vi "ReadDI.vi"(8 "error in (no error)":errorcluster, 10 "gRPCid":T5, 11 "DIOSessions In":T1={"Array of DI Sessions"=[], "Array of DO Sessions"=[], "Stream ReadDI"={"gRPCid ReadDI"=0, "DISessionName"="", "Stream Status ReadDI"=FALSE, "Async Stop ReadDI Queue"=refnum, "DI Task"="", "ms to wait"=500}}) -> (0 "error out":errorcluster, 3 "DIOSessions Out":T1={"Array of DI Sessions"=[], "Array of DO Sessions"=[], "Stream ReadDI"={"gRPCid ReadDI"=0, "DISessionName"="", "Stream Status ReadDI"=FALSE, "Async Stop ReadDI Queue"=refnum, "DI Task"="", "ms to wait"=500}})   [LabVIEW 2019, in "ctet_dio_User Library.lvlib"]
uses:
  ctet_dio_User Library.lvlib
  Servers/ctet_dio/gRPC lvSupport/Server API/typeDefs/grpcId.ctl
  Types/DIOSessions.ctl
  Types/DISession.ctl
  Types/DOSession.ctl
  Types/StreamReadDI.ctl
  Servers/ctet_dio/ctet_dio Class/RPC Messages/measurementservice_ReadDIResponse/measurementservice_ReadDIResponse_Data.ctl
  Servers/ctet_dio/ctet_dio Class/RPC Messages/measurementservice_ErrorOut/measurementservice_ErrorOut_Data.ctl
  Servers/ctet_dio/ctet_dio Class/ctet_dio.lvclass
  Servers/ctet_dio/gRPC lvSupport/gprc-lvsupport.lvlib
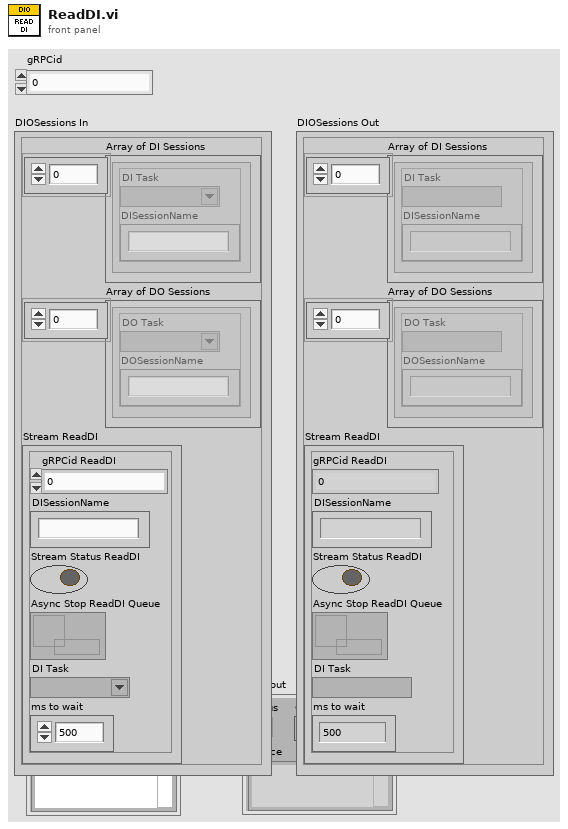
[diagram p1: front panel]
types:
  T1 = typedef "ctet_dio_User Library.lvlib/DIOSessions.ctl" = cluster{"Array of DI Sessions":T2[], "Array of DO Sessions":T3[], "Stream ReadDI":T4}
  T2 = typedef "ctet_dio_User Library.lvlib/DISession.ctl" = cluster{"DI Task":refnum<k21>, "DISessionName":string}
  T3 = typedef "ctet_dio_User Library.lvlib/DOSession.ctl" = cluster{"DO Task":refnum<k21>, "DOSessionName":string}
  T4 = typedef "ctet_dio_User Library.lvlib/StreamReadDI.ctl" = cluster{"gRPCid ReadDI":T5, "DISessionName":string, "Stream Status ReadDI":bool, "Async Stop ReadDI Queue":refnum<queue>, "DI Task":refnum<k21>, "ms to wait":u32}
  T5 = typedef "ctet_dio.lvlib/gprc-lvsupport.lvlib/grpcId.ctl" = u64
  T6 = typedef "ctet_dio.lvlib/ctet_dio.lvclass/measurementservice_ErrorOut_Data.ctl" = cluster{"errCode":i64, "errMessage":string}
  T7 = typedef "ctet_dio.lvlib/ctet_dio.lvclass/measurementservice_ReadDIResponse_Data.ctl" = cluster{"DISessionName":string, "DIData":bool[], "error":T6}
  T8 = typedef "ctet_dio.lvlib/ctet_dio.lvclass/measurementservice_ReadDIRequest_Data.ctl" = cluster{"DISessionName":string, "DISubscribeInterval":i64}
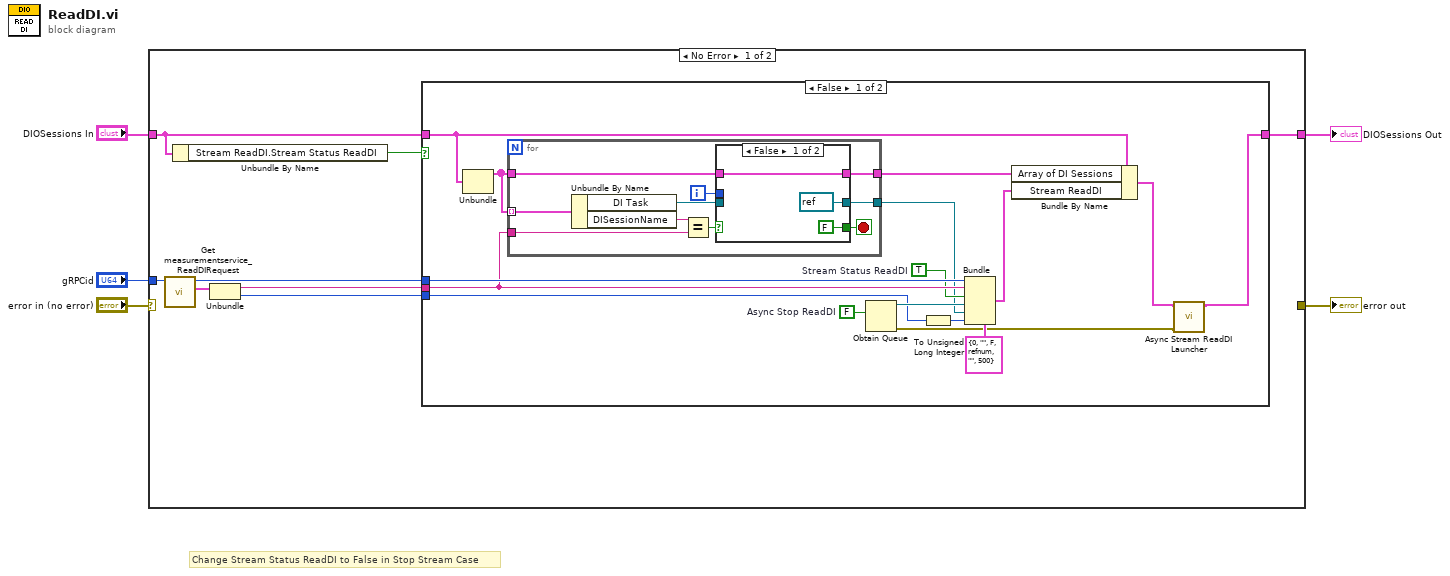
[diagram p0: block diagram]
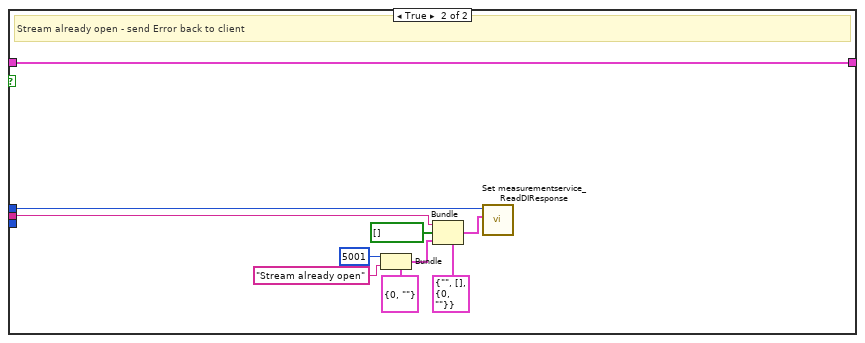
[diagram p3: hidden frame]
diagram:
  # "Change Stream Status ReadDI to False in Stop Stream Case"
  n1 = case shown="No Error" "error in (no error)" {
    selector: "error in (no error)" -> [_ w57]
    tunnel: [_ w57] -> w5
    tunnel: "gRPCid" -> [w12 _]
    tunnel: "DIOSessions In" -> [w8 w56]
    tunnel: [w13 w56] -> w1
    frame No Error {
      n2 = call "Get measurementservice_ReadDIRequest.vi"("gRPCid"=w12) -> ("Message Data"=w11:T8, "gRPCid out"=w9:T5)  [unwired: 8 in, 1 out]
      n3 = Unbundle By Name(w8) -> ("Stream ReadDI.Stream Status ReadDI"=w7:bool)
      n4 = Unbundle(w11) -> ("DISessionName"=w10:string, "DISubscribeInterval"=w6:i64)
      n5 = case shown="False" w7 {
        tunnel: [w16 w46] -> w13
        tunnel: w10 -> [w22 w52]
        tunnel: w9 -> [w26 w55]
        tunnel: w8 -> [w23 w46]
        tunnel: w6 -> [w14 _]
        frame False {
          w21 = TRUE  # Stream Status ReadDI
          w27 = FALSE  # Async Stop ReadDI
          n6 = Unbundle(w23) -> ("Array of DI Sessions"=w29:T2[])  [unwired: 2 out]
          n7 = for {
            tunnel: w29 -> [w34] mode=indexing
            tunnel: w22 -> [w39]
            tunnel: [w35] -> w19
            tunnel: w29 -> [w33]
            tunnel: [w32] -> w28
            i -> [w30]
            stop <- w37 stop-if-true
            n8 = Unbundle By Name(w34) -> ("DI Task"=w36:refnum<k21>, "DISessionName"=w31:string)
            n9 = Equal?(x=w31, y=w39) -> (x = y?=w38:bool)
            n10 = case shown="False" w38 {
              selector: w38 -> [_ w45]
              tunnel: [FALSE w45] -> w37
              tunnel: w36 -> [_ w44]
              tunnel: [refnum<k21> refnum ("DI Task") w44] -> w35
              tunnel: w33 -> [w40 w43]
              tunnel: [w40 w43] -> w32
              tunnel: w30 -> [_ _]
              frame False {
              }
              frame True {
              }
            }
          }
          n11 = Obtain Queue(element data type=w27) -> (queue out=w20:refnum<queue>, error out=w17:errorcluster)  [unwired: 4 in, 1 out]
          n12 = To Unsigned Long Integer(number=w14) -> (unsigned 32bit integer=w15:u32)
          n13 = Bundle(cluster=T4 {"gRPCid ReadDI"=0, "DISessionName"="", "Stream Status ReadDI"=FALSE, "Async Stop ReadDI Queue"=refnum, "DI Task"="", "ms to wait"=500} ("Stream ReadDI"), "gRPCid ReadDI"=w26, "DISessionName"=w22, "Stream Status ReadDI"=w21, "Async Stop ReadDI Queue"=w20, "DI Task"=w19, "ms to wait"=w15) -> (w24:T4)
          n14 = Bundle By Name(cluster=w23, "Array of DI Sessions"=w28, "Stream ReadDI"=w24) -> (w18:T1)
          n15 = call "Async Stream ReadDI Launcher.vi"("error in (no error)"=w17, "DIOSessions In"=w18) -> ("DIOSessions Out"=w16:T1)  [unwired: 8 in, 1 out]
        }
        frame True {
          # "Stream already open - send Error back to client"
          n16 = Bundle(cluster=T6 {"errCode"=0, "errMessage"=""} ("error"), "errCode"=i64 5001, "errMessage"="Stream already open") -> (w49:T6)
          n17 = Bundle(cluster=T7 {"DISessionName"="", "DIData"=[], "error"={"errCode"=0, "errMessage"=""}} ("Message Data"), "DISessionName"=w52, "DIData"=bool[] [], "error"=w49) -> (w53:T7)
          n18 = call "Set measurementservice_ReadDIResponse.vi"("Message Data"=w53, "gRPCid"=w55) -> ()  [unwired: 9 in, 1 out]
        }
      }
    }
    frame Error {
    }
  }
  "error out" <- w5
  "DIOSessions Out" <- w1
